vi "Weather Station UI.vi"(10 "하위 리미트":dbl=10.0, 11 "상위 리미트":dbl=30.0) -> (1 "경고":string, 2 "온도 히스토리":dbl(graph))   [LabVIEW 2010]
doc: "이는 기상 관측기 프로젝트의 주요 VI입니다. 온도 경고 시스템을 위한 사용자 인터페이스를 포함합니다. \n\n사용자 입력: 최대 온도, 최소 온도, 온도 단위.\n출력: 현재 온도, 경고 상태"
uses:
  Supporting Files/Weather Station States.ctl
panel:
  in  "날씨 데이터":dynamicdata(graph)
  in  "stop":bool caption="정지"
  in  "풍속 상위 리미트":dbl(slide)=50.0 scale=0.0..100.0
  out "풍속 히스토리":dbl(graph)
  # "섭씨"
  # "온도 범위"
  # "열사병"
  # "동상"
  # "kph"
  # "최대 안전 풍속"
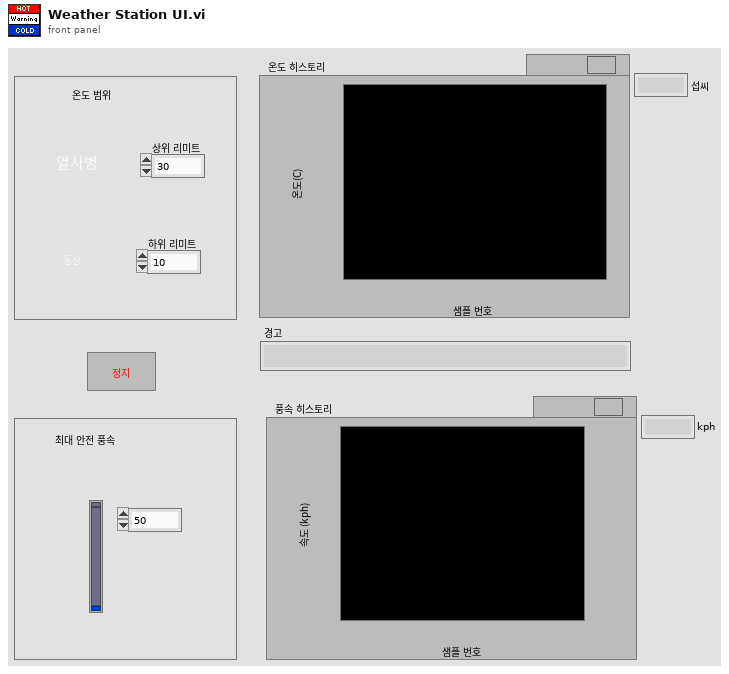
[diagram p1: front panel]
types:
  T1 = cluster{"온도":dbl, "온도 상위 리미트":dbl, "온도 하위 리미트":dbl, "풍속":dbl, "풍속 상위 리미트":dbl, "경고":string, "시간":dbl}
  T2 = typedef "Weather Station States.ctl" = enum16{"분석", "UI 처리", "경고 설정", "데이터 로그", "정지"}
  T3 = enum32{"invalid app kind", "Development System", "Run Time System", "Student Edition", "Embedded LabVIEW", "Evaluation", "Custom"}
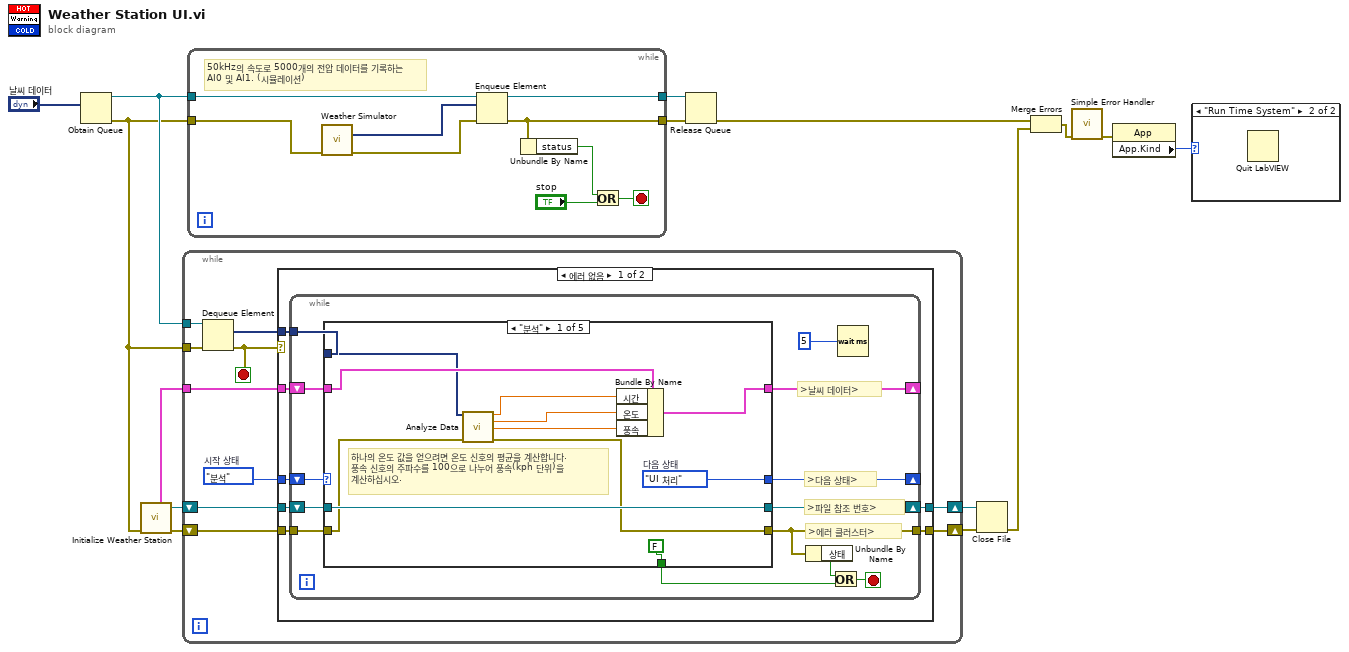
[diagram p0: block diagram]
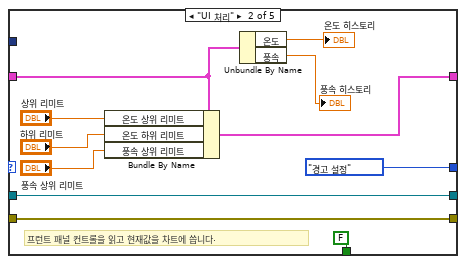
[diagram p3: hidden frame]
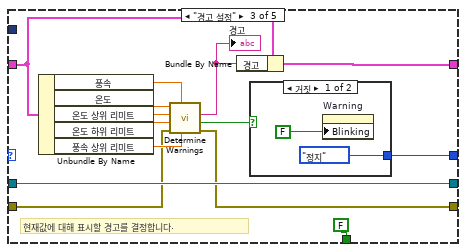
[diagram p4: hidden frame]
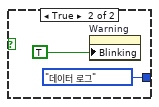
[diagram p5: hidden frame]
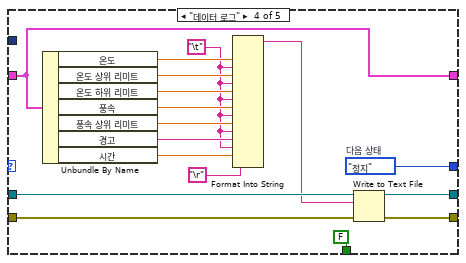
[diagram p6: hidden frame]
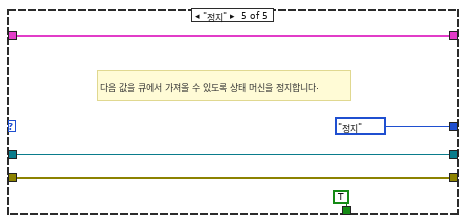
[diagram p7: hidden frame]
diagram:
  n1 = Obtain Queue(element data type="날씨 데이터") -> (queue out=w12:refnum<queue>, error out=w4:errorcluster)  [unwired: 4 in, 1 out]
  n2 = call "Initialize Weather Station.vi"("에러 입력(에러 없음)"=w4) -> ("에러 출력"=w5:cluster{"상태":bool, "코드":i32, "소스":string}, "파일 참조 번호"=w6:refnum<file>, "날씨 데이터"=w15:T1)  [unwired: 8 in]
  n3 = while {
    tunnel: w15 -> [w24]
    tunnel: w12 -> [w23]
    tunnel: w4 -> [w22]
    shift-right: [w25] -> w9
    shift-left: w6 -> [w21]
    shift-right: [w17] -> w8
    shift-left: w5 -> [w18]
    stop <- w20 stop-if-true
    w16 = Weather_Station_States."분석"  # 시작 상태
    n4 = Dequeue Element(queue=w23, error in (no error)=w22) -> (element=w19:dynamicdata, error out=w20:errorcluster)  [unwired: 1 in, 2 out]
    n5 = case shown="에러 없음" w20 {
      tunnel: [w32 w108] -> w25
      tunnel: w24 -> [w31 _]
      tunnel: w21 -> [w30 w108]
      tunnel: w19 -> [w29 _]
      tunnel: w18 -> [w27 w109]
      tunnel: [w28 w109] -> w17
      tunnel: w16 -> [w26 _]
      frame No Error {
        n6 = while {
          shift-right: [w45] -> _
          shift-left: w26 -> [w37]
          shift-right: [w35] -> w32
          shift-left: w30 -> [w44]
          shift-right: [w38] -> _
          shift-left: w31 -> [w41]
          tunnel: w29 -> [w36]
          tunnel: [w33] -> w28
          tunnel: w27 -> [w34]
          stop <- w43 stop-if-true
          # ">에러 클러스터>"
          # ">날씨 데이터>"
          # ">파일 참조 번호>"
          # ">다음 상태>"
          n7 = case shown="\"분석\"" w37 {
            tunnel: [w56 Weather_Station_States."경고 설정" ("Next State") w80 w102 Weather_Station_States."정지" ("Next State")] -> w45
            tunnel: [w46 w58 w70 w99 w103] -> w33
            tunnel: w44 -> [w52 w57 w77 w98 w104]
            tunnel: [w53 w67 w78 w96 w105] -> w38
            tunnel: w41 -> [w54 w64 w79 w96 w105]
            tunnel: [FALSE ("stop") FALSE ("stop") FALSE ("stop") FALSE ("stop") TRUE ("stop")] -> w40
            tunnel: w36 -> [w51 _ _ _ _]
            tunnel: [w52 w57 w77 w100 w104] -> w35
            tunnel: w34 -> [w50 w58 w71 w86 w103]
            frame "분석" {
              w56 = Weather_Station_States."UI 처리"  # 다음 상태
              # "하나의 온도 값을 얻으려면 온도 신호의 평균을 계산합니다. 풍속 신호의 주파수를 100으로 나누어 풍속(kph 단위)을 계산하십시오."
              n8 = call "Analyze Data.vi"("날씨 데이터"=w51, "에러 입력"=w50) -> ("시간"=w49:dbl, "온도"=w48:dbl, "풍속"=w47:dbl, "에러 출력"=w46:errorcluster)  [unwired: 10 in]
              n9 = Bundle By Name(cluster=w54, "시간"=w49, "온도"=w48, "풍속"=w47) -> (w53:T1)
            }
            frame "UI 처리" {
              # "프런트 패널 컨트롤을 읽고 현재값을 차트에 씁니다."
              n10 = Bundle By Name(cluster=w64, "온도 상위 리미트"="상위 리미트", "온도 하위 리미트"="하위 리미트", "풍속 상위 리미트"="풍속 상위 리미트") -> (w67:T1)
              n11 = Unbundle By Name(w64) -> ("온도"=→"온도 히스토리":dbl, "풍속"=→"풍속 히스토리":dbl)
            }
            frame "경고 설정" {
              # "현재값에 대해 표시할 경고를 결정합니다."
              n12 = Unbundle By Name(w79) -> ("풍속"=w76:dbl, "온도"=w75:dbl, "온도 상위 리미트"=w74:dbl, "온도 하위 리미트"=w73:dbl, "풍속 상위 리미트"=w72:dbl)
              n13 = call "Determine Warnings.vi"("최대 풍속"=w72, "현재 풍속"=w76, "에러 입력(에러 없음)"=w71, "최저 온도"=w73, "최고 온도"=w74, "현재 온도"=w75) -> ("에러 없음"=w70:errorcluster, "경고?"=w69:bool, "경고 텍스트"=w68:string)  [unwired: 3 in]
              "경고" <- w68
              n14 = Bundle By Name(cluster=w79, "경고"=w68) -> (w78:T1)
              n15 = case shown="거짓" w69 {
                tunnel: [Weather_Station_States."정지" ("Next State") Weather_Station_States."데이터 로그" ("Next State")] -> w80
                frame False {
                  n16 = property on="Warning" class="Str"("Blinking"=FALSE) -> ()  [unwired: 2 in, 2 out]
                }
                frame True {
                  n17 = property on="Warning" class="Str"("Blinking"=TRUE) -> ()  [unwired: 2 in, 2 out]
                }
              }
            }
            frame "데이터 로그" {
              w88 = "\t"
              w102 = Weather_Station_States."정지"  # 다음 상태
              n18 = Unbundle By Name(w96) -> ("온도"=w95:dbl, "온도 상위 리미트"=w94:dbl, "온도 하위 리미트"=w93:dbl, "풍속"=w92:dbl, "풍속 상위 리미트"=w91:dbl, "경고"=w90:string, "시간"=w89:dbl)
              n19 = Format Into String(w95, w88, w94, w88, w93, w88, w92, w88, w91, w88, w90, w88, w89, "\r") -> (resulting string=w97:string)  [unwired: 3 in, 1 out]
              n20 = Write to Text File(file (use dialog)=w98, text=w97, error in=w86) -> (refnum out=w100:refnum<file>, error out=w99:errorcluster)  [unwired: 1 in, 1 out]
            }
            frame "정지" {
              # "다음 값을 큐에서 가져올 수 있도록 상태 머신을 정지합니다."
            }
          }
          n21 = Unbundle By Name(w33) -> ("상태"=w42:bool)
          n22 = Or(x=w42, y=w40) -> (x .or. y?=w43:bool)
          n23 = Wait (ms)(milliseconds to wait=u32 5 ("y")) -> ()  [unwired: 1 out]
        }
      }
      frame Error {
      }
    }
  }
  n24 = while {
    tunnel: w12 -> [w118]
    tunnel: w4 -> [w112]
    tunnel: [w115] -> w14
    tunnel: [w117] -> w13
    stop <- w113 stop-if-true
    # "50kHz의 속도로 5000개의 전압 데이터를 기록하는 AI0 및 AI1. (시뮬레이션)"
    n25 = call "Weather Simulator.vi"("에러 입력(에러 없음)"=w112) -> ("웨이브폼 그래프"=w110:dynamicdata, "에러 출력"=w111:errorcluster)  [unwired: 13 in]
    n26 = Enqueue Element(queue=w118, element=w110, error in (no error)=w111) -> (queue out=w117:refnum<queue>, error out=w115:errorcluster)  [unwired: 1 in, 1 out]
    n27 = Unbundle By Name(w115) -> ("status"=w114:bool)
    n28 = Or(x=w114, y="stop") -> (x .or. y?=w113:bool)
  }
  n29 = Release Queue(queue=w13, error in (no error)=w14) -> (error out=w1:errorcluster)  [unwired: 1 in, 2 out]
  n30 = Close File(refnum=w9, error in=w8) -> (error out=w7:errorcluster)  [unwired: 1 out]
  n31 = Merge Errors(w1, w7) -> (w10:errorcluster)
  n32 = call <vilib>:"Simple Error Handler.vi"("error in (no error)"=w10) -> ("error out"=w2:errorcluster)  [unwired: 4 in, 4 out]
  n33 = property class="App"(error in=w2) -> ("App.Kind"=w3:T3)  [unwired: 1 in, 2 out]
  n34 = case shown="\"Run Time System\"" w3 {
    frame "invalid app kind", Default {
    }
    frame "Run Time System" {
      n35 = Quit LabVIEW() -> ()  [unwired: 1 in]
    }
  }
